vi "tree select mouse down action.vi"(8 "error in (no error)":errorcluster, 10 "Mouse down data":T1, 11 "Loop data":T2) -> (0 "error out":errorcluster, 2 "New Selection states":bool[](array[boolean]), 3 "Loop data":T2)   [LabVIEW 2020, in "UI_ItemSelect.lvlib"]
uses:
  UI_ItemSelect.lvlib
  Tree item select loop data.ctl
  Item select ref type.ctl
  Tree item loop data.ctl
  Tree item selection indices.ctl
  checkbox state.ctl
  item select tree lock states.ctl
  item select mouse down data.ctl
  item select calc action.ctl
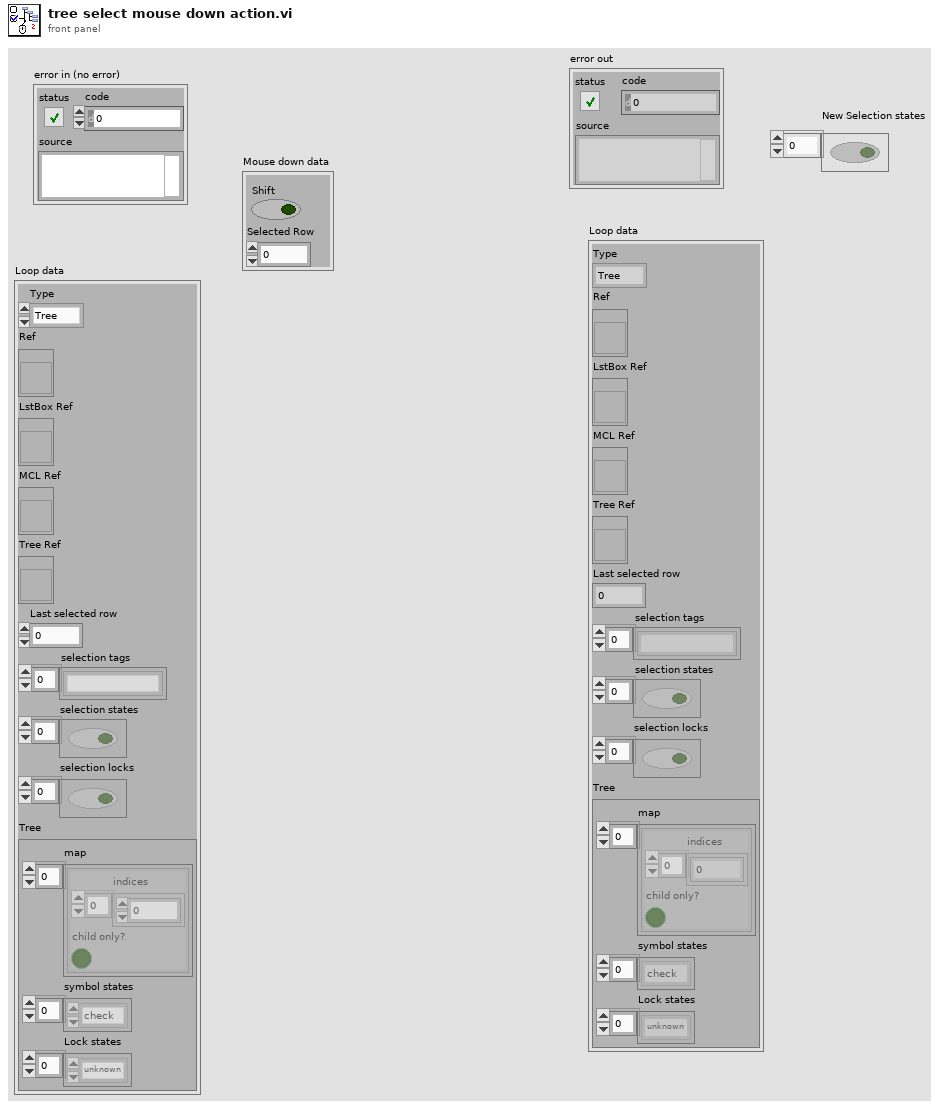
[diagram p1: front panel]
types:
  T1 = typedef "UI_ItemSelect.lvlib/item select mouse down data.ctl" = cluster{"Shift":bool, "Selected Row":i32}
  T2 = typedef "UI_ItemSelect.lvlib/Tree item select loop data.ctl" = cluster{"Type":T3, "Ref":refnum<vi>, "LstBox Ref":refnum<vi>, "MCL Ref":refnum<vi>, "Tree Ref":refnum<vi>, "Last selected row":i32, "selection tags":string[], "selection states":bool[], "selection locks":bool[], "Tree":T4}
  T3 = typedef "UI_ItemSelect.lvlib/Item select ref type.ctl" = enum16{"Tree", "MCL", "ListBox"}
  T4 = typedef "UI_ItemSelect.lvlib/Tree item loop data.ctl" = cluster{"map":T5[], "symbol states":T6[], "Lock states":T7[]}
  T5 = typedef "UI_ItemSelect.lvlib/Tree item selection indices.ctl" = cluster{"indices":i32[], "child only?":bool}
  T6 = typedef "UI_ItemSelect.lvlib/checkbox state.ctl" = enum16{"unknown", "check", "some", "no check"}
  T7 = typedef "UI_ItemSelect.lvlib/item select tree lock states.ctl" = enum16{"unknown", "locked", "unlocked"}
  T8 = typedef "UI_ItemSelect.lvlib/item select calc action.ctl" = enum16{"false", "true", "invert"}
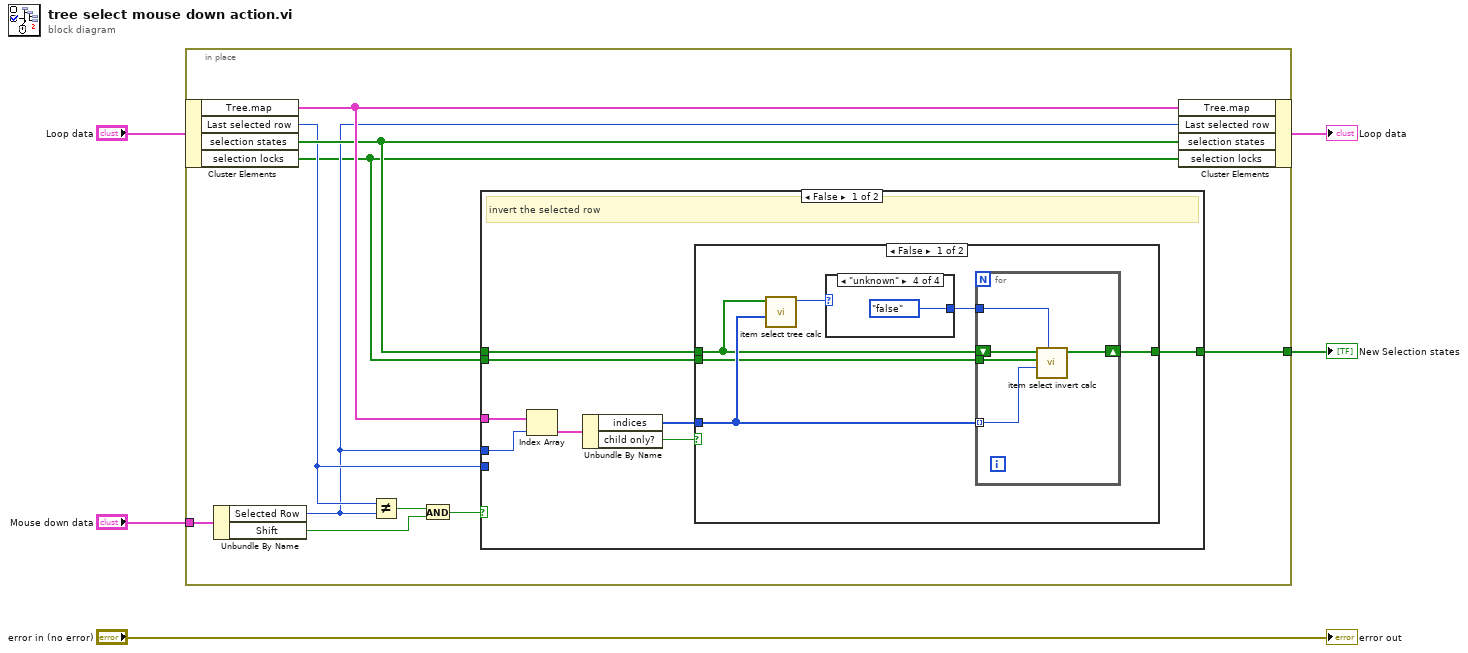
[diagram p0: block diagram]
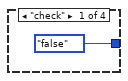
[diagram p2: hidden frame]
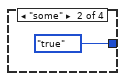
[diagram p3: hidden frame]
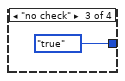
[diagram p4: hidden frame]
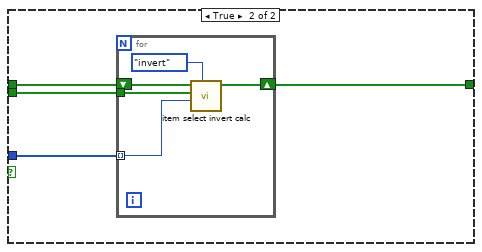
[diagram p5: hidden frame]
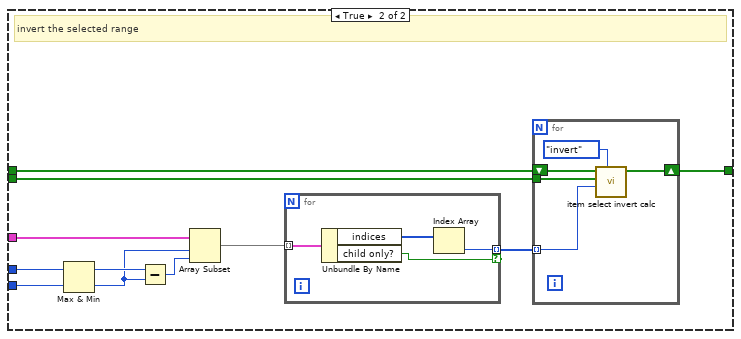
[diagram p6: hidden frame]
diagram:
  n1 = in-place {
    in-place-border: "Mouse down data" -> [w15]
    in-place-border: [w12] -> w3
    n2 = in-place-cluster #1("Loop data") -> ("Tree.map"=w14:T5[], "Last selected row"=w10:i32, "selection states"=w13:bool[], "selection locks"=w6:bool[])
    n3 = Unbundle By Name(w15) -> ("Selected Row"=w9:i32, "Shift"=w8:bool)
    n4 = Not Equal?(x=w10, y=w9) -> (x != y?=w11:bool)
    n5 = And(x=w11, y=w8) -> (x .and. y?=w7:bool)
    n6 = case shown="False" w7 {
      tunnel: w9 -> [w22 w58]
      tunnel: w10 -> [_ w57]
      tunnel: w14 -> [w23 w56]
      tunnel: w13 -> [w20 w51]
      tunnel: [w18 w49] -> w12
      tunnel: w6 -> [w21 w48]
      frame False {
        # "invert the selected row"
        n7 = Index Array(array=w23, index=w22) -> (element=w19:T5)
        n8 = Unbundle By Name(w19) -> ("indices"=w17:i32[], "child only?"=w16:bool)
        n9 = case shown="False" w16 {
          tunnel: w21 -> [w27 w42]
          tunnel: w20 -> [w28 w41]
          tunnel: [w26 w40] -> w18
          tunnel: w17 -> [w29 w39]
          frame False {
            n10 = call "item select tree calc.vi"("indices"=w29, "selection states"=w28) -> ("symbol state"=w25:T6)  [unwired: 9 in]
            n11 = case shown="\"unknown\"" w25 {
              tunnel: [item_select_calc_action."false" ("Action") item_select_calc_action."true" ("Action") item_select_calc_action."true" ("Action") item_select_calc_action."false" ("Action")] -> w24
              frame "check" {
              }
              frame "some" {
              }
              frame "no check" {
              }
              frame "unknown" {
              }
            }
            n12 = for {
              tunnel: w29 -> [w36] mode=indexing
              shift-right: [w35] -> w26
              shift-left: w28 -> [w38]
              tunnel: w27 -> [w37]
              tunnel: w24 -> [w34]
              n13 = call "item select invert calc.vi"("Action"=w34, "selection index"=w36, "selection locks"=w37, "selection states"=w38) -> ("new selection states"=w35:bool[])  [unwired: 7 in]
            }
          }
          frame True {
            n14 = for {
              tunnel: w42 -> [w46]
              tunnel: w39 -> [w45] mode=indexing
              shift-right: [w44] -> w40
              shift-left: w41 -> [w47]
              n15 = call "item select invert calc.vi"("Action"=item_select_calc_action."invert", "selection index"=w45, "selection locks"=w46, "selection states"=w47) -> ("new selection states"=w44:bool[])  [unwired: 7 in]
            }
          }
        }
      }
      frame True {
        # "invert the selected range"
        n16 = Max & Min(x=w58, y=w57) -> (max(x,y)=w55:i32, min(x,y)=w54:i32)
        n17 = Subtract(x=w55, y=w54) -> (x-y=w53:i32)
        n18 = Array Subset(array=w56, index=w54, length=w53) -> (w52:T5[])
        n19 = for {
          tunnel: w52 -> [w62] mode=indexing
          tunnel: [w60] -> w50 mode=indexing if=w59
          n20 = Unbundle By Name(w62) -> ("indices"=w61:i32[], "child only?"=w59:bool)
          n21 = Index Array(array=w61) -> (element=w60:i32)  [unwired: 1 in]
        }
        n22 = for {
          tunnel: w50 -> [w65] mode=indexing
          shift-right: [w64] -> w49
          shift-left: w51 -> [w67]
          tunnel: w48 -> [w66]
          n23 = call "item select invert calc.vi"("Action"=item_select_calc_action."invert", "selection index"=w65, "selection locks"=w66, "selection states"=w67) -> ("new selection states"=w64:bool[])  [unwired: 7 in]
        }
      }
    }
    n24 = in-place-cluster #1("Tree.map"=w14, "Last selected row"=w9, "selection states"=w13, "selection locks"=w6) -> (→"Loop data":T2)
  }
  "New Selection states" <- w3
  "error out" <- "error in (no error)"
